vi "xml.boolean.vi"(10 "Value":variant, 11 "MsgSerializer.XML in":refnum<class "MsgSerializer.XML.lvclass">) -> (3 "string":string)   [LabVIEW 2020, in "Caraya.lvlib" / "MsgSerializer.XML.lvclass"]
uses:
  MsgSerializer.XML.lvclass
  C:/projects/caraya/src/classes/MsgSerializer/MsgSerializer.lvclass
  MsgSerializer.XML.lvclass/MsgSerializer.XML.ctl
  MsgSerializer/MsgSerializer.lvclass/MsgSerializer.ctl
  MsgSerializer/MsgSerializer.lvclass
  <vilib>/Utility/VariantDataType/VariantType.lvlib
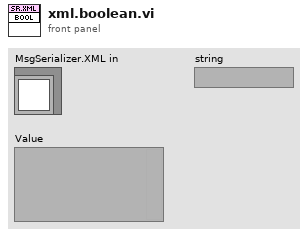
[diagram p1: front panel]
types:
  T1 = typedef "VariantType.lvlib/Type.ctl" = enum8{"Invalid Type", "Void", "I8", "I16", "I32", "I64", "U8", "U16", "U32", "U64", "Single Float", "Double Float", "Extended Float", "Single Complex", "Double Complex", "Extended Complex", "Enum U8", "Enum U16", "Enum U32", "Enum U64", "Single Float With Unit", "Double Float With Unit", "Extended Float With Unit", "Single Complex with Unit", "Double Complex with Unit", "Extended Complex with Unit", "Boolean", "String", "Path", "Picture", "Tag", "Array", "Cluster", "Variant", "LV Variant", "Waveform", "Timestamp", "Digital Waveform", "Digital Data", "ExpressData", "Refnum", "External Data", "VI", "Poly VI", "LabVIEW Class Instance", "Fixed Point"}
  T2 = typedef "Caraya.lvlib/MsgSerializer.XML.lvclass/format -- enum.ctl" = enum16{"value", "tag", "property"}
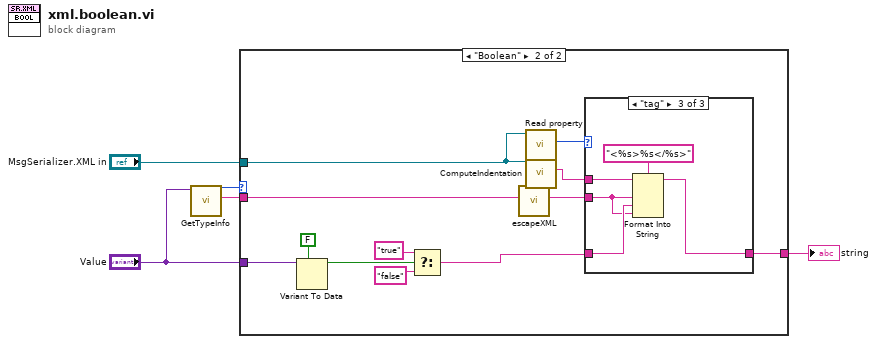
[diagram p0: block diagram]
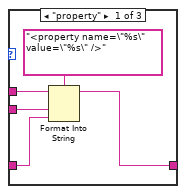
[diagram p3: hidden frame]
diagram:
  n1 = call <vilib>:"GetTypeInfo.vi"("Variant"="Value") -> ("Name"=w4:string, "Type Enum"=w1:T1)  [unwired: 6 in, 3 out]
  n2 = case shown="\"Boolean\"" w1 {
    tunnel: "Value" -> [_ w7]
    tunnel: w4 -> [_ w15]
    tunnel: "MsgSerializer.XML in" -> [_ w13]
    tunnel: [_ w12] -> w2
    frame Default {
    }
    frame "Boolean" {
      n3 = Variant To Data(type=FALSE, Variant=w7) -> (data=w8:bool)  [unwired: 1 in, 1 out]
      n4 = Select(t="true", s=w8, f="false") -> (s? t:f=w6:string)
      n5 = call "escapeXML.vi"("Input String"=w15) -> ("XML-escaped String"=w16:string)  [unwired: 10 in]
      n6 = call "Read property.vi"("MsgSerializer.XMLProperty in"=w13) -> ("format"=w17:T2)  [unwired: 9 in, 1 out]
      n7 = call "ComputeIndentation.vi"("MsgSerializer in"=w13) -> ("indentation"=w14:string)  [unwired: 10 in]
      n8 = case shown="\"tag\"" w17 {
        tunnel: w6 -> [w21 w23 w27]
        tunnel: [w20 w23 w24] -> w12
        tunnel: w14 -> [w18 _ w26]
        tunnel: w16 -> [w19 _ w25]
        frame "property" {
          n9 = Format Into String(format string="<property name=\"%s\" value=\"%s\" />" ("name"), initial string=w18, w19, w21) -> (resulting string=w20:string)  [unwired: 1 in, 1 out]
        }
        frame "value" {
        }
        frame "tag" {
          n10 = Format Into String(format string="<%s>%s</%s>" ("name"), initial string=w26, w25, w27, w25) -> (resulting string=w24:string)  [unwired: 1 in, 1 out]
        }
      }
    }
  }
  "string" <- w2
